vi "Kinimatics_Matrix_SetRow.vi"(9 "Fill Row Vector":T1, 10 "Row":i32, 11 "input matrix":T1) -> (0 "Error":bool, 3 "output matrix":T1)   [LabVIEW 2023, in "Swerve_Odometry_SEN.lvlib"]
doc: "Sets a row to a given row vector.\n \n\nInputs:\n - input matrix -- The input matrix\n - row -- The row to set.\n - val -- The row vector to set the given row to.\n\nOutputs:\n - output matrix -- resulting matrix\n - error -- If TRUE, an error occured."
uses:
  Swerve_Odometry_SEN.lvlib
  <vilib>/Analysis/Matrix/Datatypes/RealMatrix.ctl
  <vilib>/Analysis/Matrix/NI_Matrix.lvlib
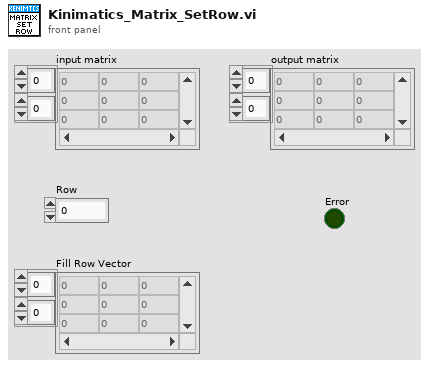
[diagram p1: front panel]
types:
  T1 = typedef "NI_Matrix.lvlib/RealMatrix.ctl" = dbl[][]
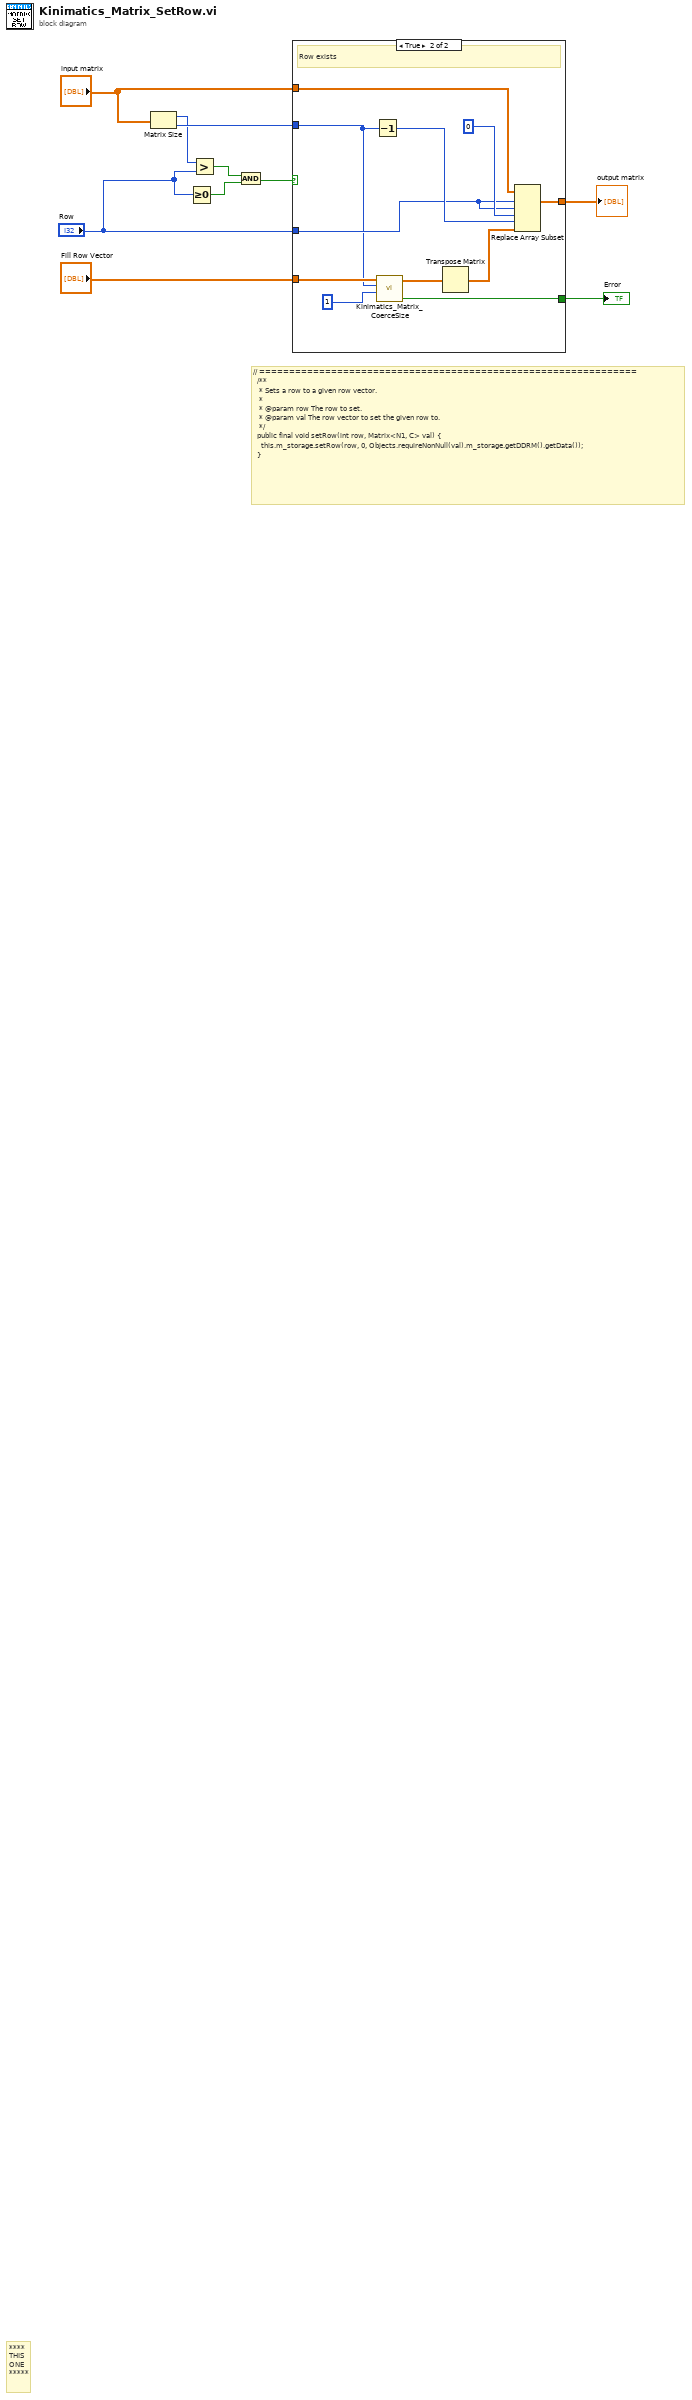
[diagram p0: block diagram]
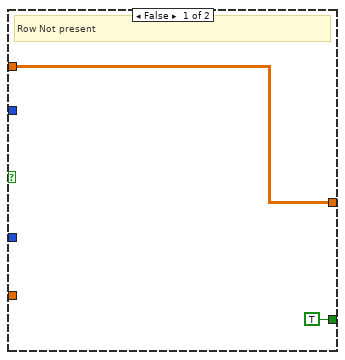
[diagram p2: hidden frame]
diagram:
  # "// ===============================================================\n  /**\n   * Sets a row to a given row vector.\n   *\n   * @param row The row to set.\n   * @param val The row vector to set the given row to.\n   */\n  public final void setRow(int row, Matrix<N1, C> val) {\n    this.m_storage.setRow(row, 0, Objects.requireNonNull(val).m_storage.getDDRM().getData());\n  }"
  # "****\nTHIS\nONE\n*****"
  n1 = Matrix Size(0:"input matrix") -> (1:w4:i32, 2:w7:i32)
  n2 = Greater Or Equal To 0?(x="Row") -> (x >= 0?=w5:bool)
  n3 = Greater?(x=w4, y="Row") -> (0:w6:bool)
  n4 = And(x=w6, y=w5) -> (x .and. y?=w1:bool)
  n5 = case shown="True" w1 {
    tunnel: "Fill Row Vector" -> [_ w23]
    tunnel: "input matrix" -> [w11 w22]
    tunnel: [w11 w21] -> w8
    tunnel: w7 -> [_ w16]
    tunnel: "Row" -> [_ w18]
    tunnel: [TRUE ("Coerced") w17] -> w2
    frame False {
      # "Row Not present"
    }
    frame True {
      # "Row exists"
      n6 = Decrement(x=w16) -> (x-1=w19:i32)
      n7 = call "Kinimatics_Matrix_CoerceSize.vi"("Columns"=1, "Rows"=w16, "input matrix"=w23) -> ("Coerced"=w17:bool, "output matrix"=w14:T1)  [unwired: 7 in]
      n8 = Transpose Matrix(1:w14) -> (0:w13:T1)
      n9 = Replace Array Subset(array=w22, new element=w13, index (dim 0)=w18, index (dim 1)=w18, index (dim 2)=0 ("row 1"), index (dim 3)=w19) -> (w21:T1)
    }
  }
  "output matrix" <- w8
  "Error" <- w2
